vi "Grab TCP Status Data.vi"(0 "connection ID":refnum<k5>, 1 "No timeout?":bool, 3 "error in (no error)":errorcluster) -> (7 "Status ID out":refnum<k5>, 8 "data out":string, 10 "error out":errorcluster)   [LabVIEW 2015]
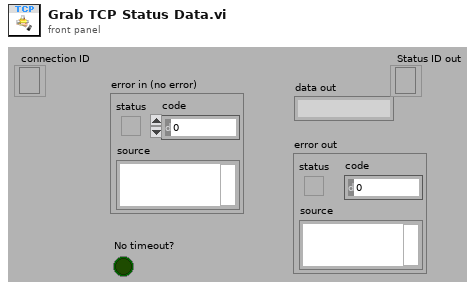
[diagram p1: front panel]
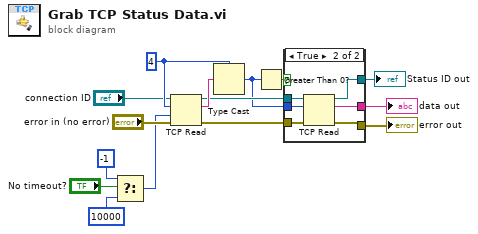
[diagram p0: block diagram]
diagram:
  w9 = 4
  n1 = Select(t=-1 ("timeout ms (25000)"), s="No timeout?", f=10000 ("timeout ms (25000)")) -> (s? t:f=w4:i32)
  n2 = TCP Read(connection ID="connection ID", bytes to read=w9, error in (no error)="error in (no error)", 9:w4) -> (connection ID out=w11:refnum<k5>, data out=w12:string, error out=w10:errorcluster)  [unwired: 1 in]
  n3 = Type Cast(type=w9, x=w12) -> (*(type *) &x=w7:i32)
  n4 = Greater Than 0?(x=w7) -> (x > 0?=w8:bool)
  n5 = case shown="True" w8 {
    tunnel: [_ w23] -> w15
    tunnel: [w16 w22] -> w14
    tunnel: w11 -> [w17 w21]
    tunnel: w10 -> [w16 w20]
    tunnel: w7 -> [_ w18]
    tunnel: [w17 w19] -> w2
    frame False {
    }
    frame True {
      n6 = TCP Read(connection ID=w21, bytes to read=w18, error in (no error)=w20) -> (connection ID out=w19:refnum<k5>, data out=w23:string, error out=w22:errorcluster)  [unwired: 2 in]
    }
  }
  "data out" <- w15
  "error out" <- w14
  "Status ID out" <- w2
